vi "Cluster operazioni.vi"() -> ()   [LabVIEW 2012]
panel:
  out "Cluster":cluster{"Numeric":dbl, "Boolean":bool} {"Numeric" format="%.2f"}
  out "data clst 2":T1={"txt "="", "index "=4, "data "=0.0, "valid "=FALSE} {"data" format="%.1f"}
  out "data sel":sgl format="%.1f"
  out "txt sel":string
  in  "valid":bool
  in  "value":sgl=1.0 format="%.1f"
  in  "position":i32=4
  in  "type":string="temp"
  out "valid":bool
  out "data":sgl format="%.1f"
  out "index":i32=4
  out "txt":string
  out "data clst":T2={"txt"="", "index "=4, "data "=0.0, "valid "=FALSE} {"data" format="%.1f"}
  # "Funzioni che operano sui clusters"
  # "Bundle"
  # "Unbundle"
  # "Bundle By Name"
  # "Unbundle By Name"
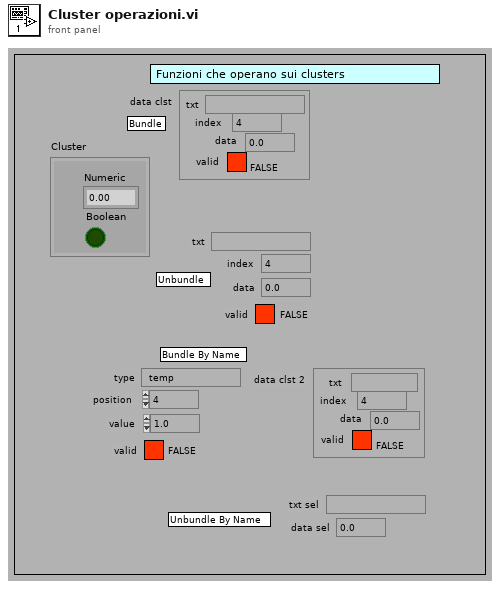
[diagram p1: front panel]
types:
  T1 = cluster{"txt ":string, "index ":i32, "data ":sgl, "valid ":bool}
  T2 = cluster{"txt":string, "index ":i32, "data ":sgl, "valid ":bool}
  T3 = cluster{"txt":string, "index":i32, "data":sgl, "valid":bool}
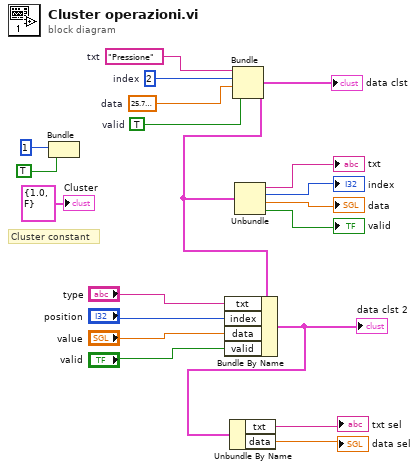
[diagram p0: block diagram]
diagram:
  w18 = sgl 25.7  # data
  w17 = TRUE  # valid
  w19 = "Pressione"  # txt
  w5 = 2  # index
  # "Cluster constant"
  n1 = Bundle(1, TRUE) -> ()  [unwired: 1 in, 1 out]
  n2 = Bundle "Bundle"("txt"=w19, "index"=w5, "data"=w18, "valid"=w17) -> (w11:T3)  [unwired: 1 in]
  "data clst" <- w11
  n3 = Bundle By Name "Bundle By Name"(cluster=w11, "txt"="type", "index"="position", "data"="value", "valid"="valid") -> (w4:T3)
  "data clst 2" <- w4
  n4 = Unbundle By Name "Unbundle By Name"(w4) -> ("txt"=→"txt sel":string, "data"=→"data sel":sgl)
  n5 = Unbundle "Unbundle"(w11) -> ("txt"=→"txt":string, "index"=→"index":i32, "data"=→"data":sgl, "valid"=→"valid":bool)
  "Cluster" <- cluster{"Numeric":dbl, "Boolean":bool} {"Numeric"=1.0, "Boolean"=FALSE} ("Cluster")
